vi "Write Object Bytes.vi"(8 "Error In":errorcluster) -> (0 "Error Out":errorcluster)   [LabVIEW 2018, in "Tests.lvlib" / "Writer.lvlib"]
uses:
  Writer.lvlib
  src/Toolkit/Public/Writer/Writer.lvclass/Writer.ctl
  src/Toolkit/Public/Writer/Private/Handle Error.vi
  src/Toolkit/Public/Writer/Public/Status/Read Is Error.vi
  src/Toolkit/Public/Writer/Public/Status/Read Status.vi
  src/Toolkit/Public/Writer/Public/Status/Read Status Message.vi
  src/Toolkit/Public/Utility/Status Code.vi
  <vilib>/Utility/error.llb/Error Cluster From Error Code.vi
  <vilib>/addons/_JKI Toolkits/Caraya/classes/Test/Test.lvclass
  <vilib>/addons/_JKI Toolkits/Caraya/classes/Assert/Assert.lvclass
  src/Toolkit/Public/Writer/Writer.lvclass
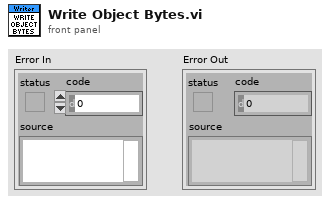
[diagram p1: front panel]
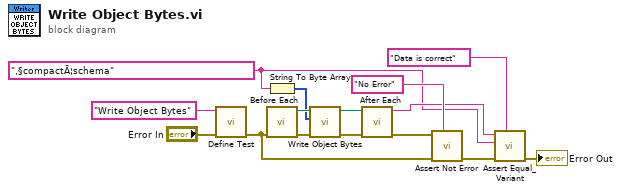
[diagram p0: block diagram]
diagram:
  w1 = "‚§compactÃ¦schema" ("Data")
  n1 = call <vilib>:"Define Test.vi"("error in (no error)"="Error In", "Label (VI Title)"="Write Object Bytes") -> ("error out"=w11:errorcluster)  [unwired: 9 in]
  n2 = String To Byte Array(string=w1) -> (unsigned byte array=w2:u8[])
  n3 = call "Before Each.vi"("Error In"=w11) -> ("Error Out"=w7:errorcluster, "Writer Out"=w6:refnum<class "Writer.lvclass">)  [unwired: 9 in]
  n4 = call "Write Object Bytes.vi"("Error In"=w7, "Value"=w2, "Writer In"=w6) -> ("Error Out"=w4:errorcluster, "Writer Out"=w5:refnum<class "Writer.lvclass">)  [unwired: 7 in]
  n5 = call "After Each.vi"("Error In"=w4, "Writer In"=w5) -> ("Error Out"=w10:errorcluster, "Data"=w3:string)  [unwired: 8 in]
  n6 = call <vilib>:"Assert Not Error.vi"("Label"="No Error", "error in (no error)"=w11, "Not Error?"=w10) -> ("error out"=w13:errorcluster)  [unwired: 8 in]
  n7 = call <vilib>:"Assert Equal_Variant.vi"("Label"="Data is correct", "error in (no error)"=w13, "Y"=w1, "X"=w3) -> ("error out"=→"Error Out":errorcluster)  [unwired: 7 in]
